vi "外观 1.vi"(0 "Data In":T8 caption="数据输入", 2 "Display State In":T6 caption="显示状态输入", 3 "Container State":T7 caption="容器状态") -> (6 "Data Out":T8 caption="数据输出", 7 "Display State Out":T6 caption="显示状态输出", 8 "Action":T5 caption="动作")   [LabVIEW 2013, in "Bit by Bit Adjust_Xcontrol.xctl"]
uses:
  Bit by Bit Adjust_Xcontrol.xctl
  <vilib>/_xctls/Container State.ctl
  <vilib>/_xctls/Action.ctl
  Bit_Display.ctl
  Up_Key.ctl
  Down_Key.ctl
  %_Display.ctl
  <vilib>/_xctls/XControlSupport.lvlib
panel:
  out "Totol Number":i32
  in  "Zero":bool
  out "小数点":bool=TRUE
  out "字符串":T1="%"
  in  "Down_x1":T2
  in  "Down_x10":T2
  in  "Down_x100":T2
  in  "Down_x1000":T2
  in  "Up_x1":T3
  in  "Up_x10":T3
  in  "Up_x100":T3
  in  "Up_x1000":T3
  out "Str_x1":T4="0"
  out "Str_x10":T4="0"
  out "Str_x100":T4="0"
  out "Str_x1000":T4="0"
  in  "Down_x10000":T2
  in  "Up_x10000":T3
  out "Str_x10000":T4="0"
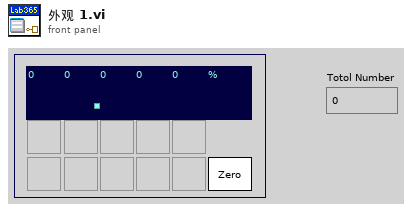
[diagram p1: front panel]
types:
  T1 = typedef "%_Display.ctl" = string
  T2 = typedef "Down_Key.ctl" = bool
  T3 = typedef "Up_Key.ctl" = bool
  T4 = typedef "Bit_Display.ctl" = string
  T5 = typedef "XControlSupport.lvlib/Action.ctl" = cluster{"Data Changed?":bool, "State Changed?":bool, "Action Name":string}
  T6 = typedef "Bit by Bit Adjust_Xcontrol.xctl/状态 1.ctl" = cluster{"Numeric":dbl}
  T7 = typedef "XControlSupport.lvlib/Container State.ctl" = cluster{"Indicator?":bool, "Run Mode?":bool, " Refnum":refnum<vi>}
  T8 = typedef "Bit by Bit Adjust_Xcontrol.xctl/数据 1.ctl" = dbl
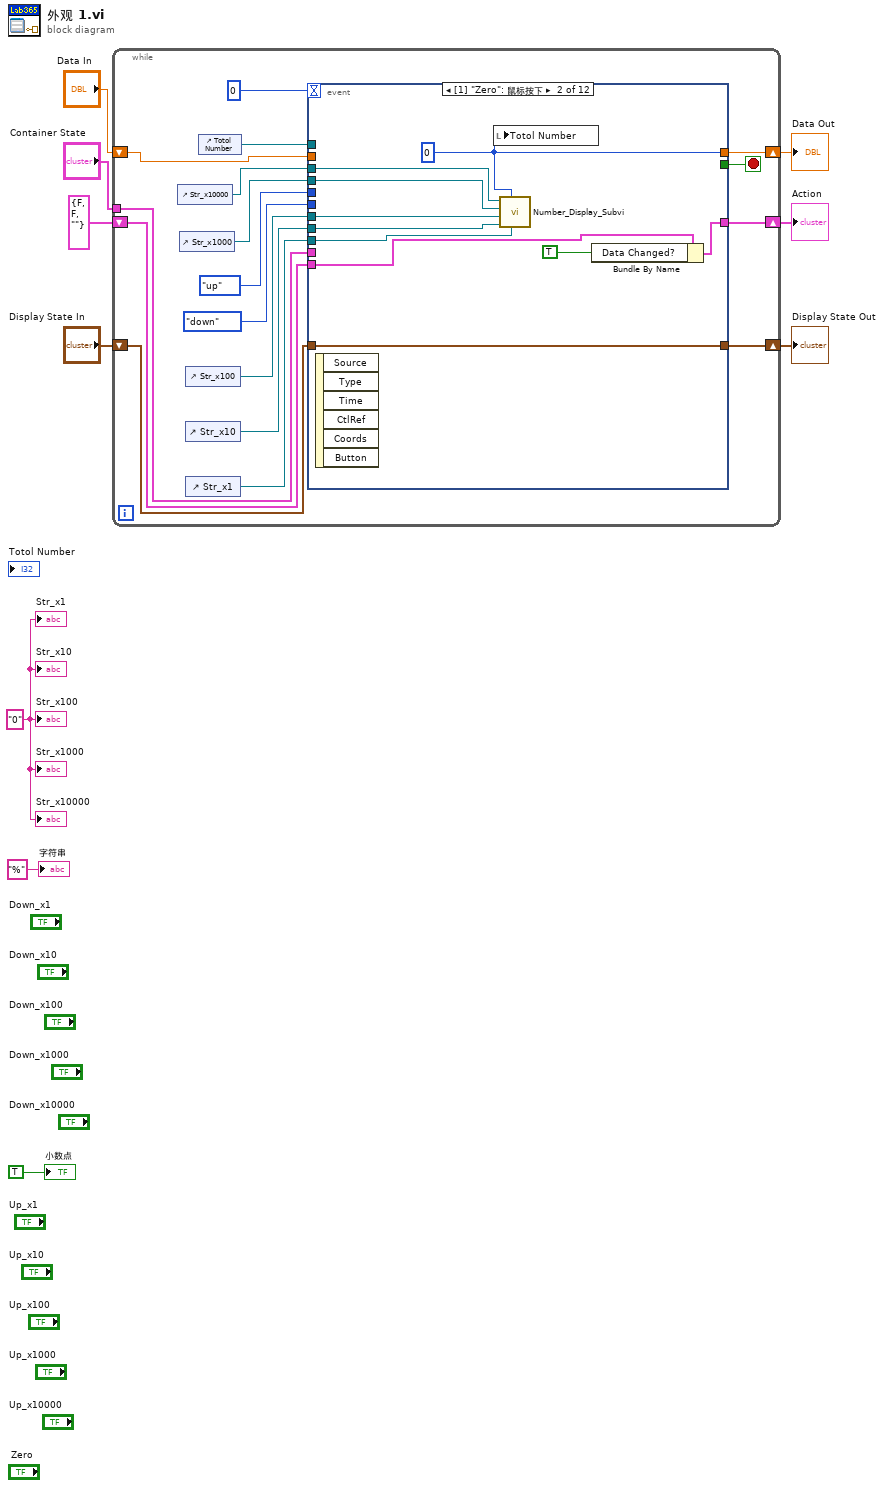
[diagram p0: block diagram]
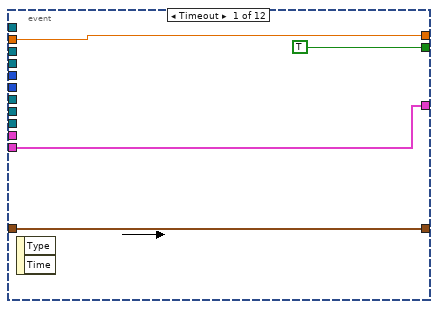
[diagram p2: hidden frame]
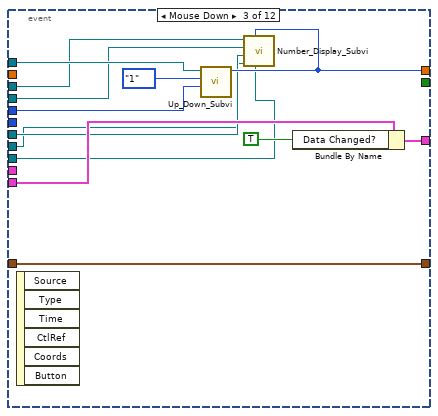
[diagram p3: hidden frame]
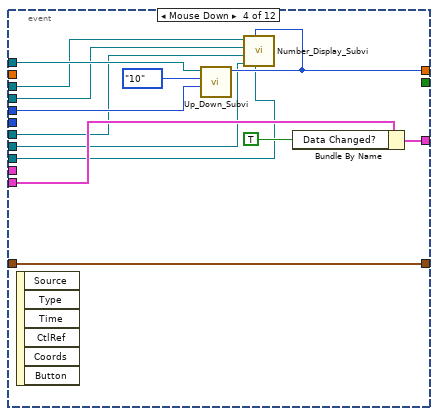
[diagram p4: hidden frame]
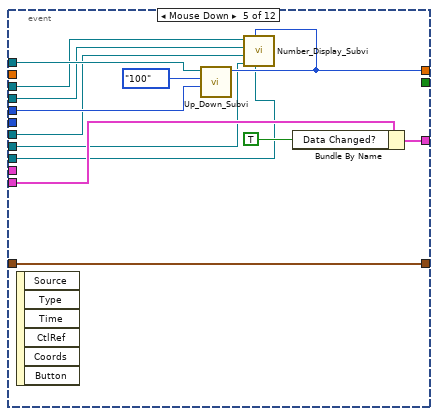
[diagram p5: hidden frame]
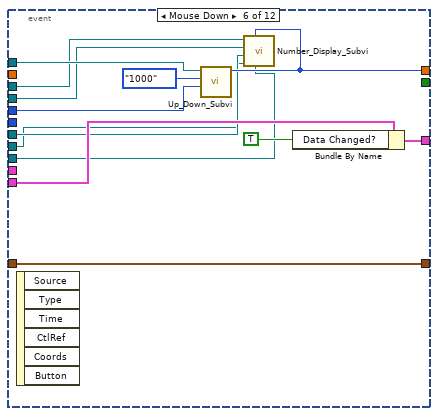
[diagram p6: hidden frame]
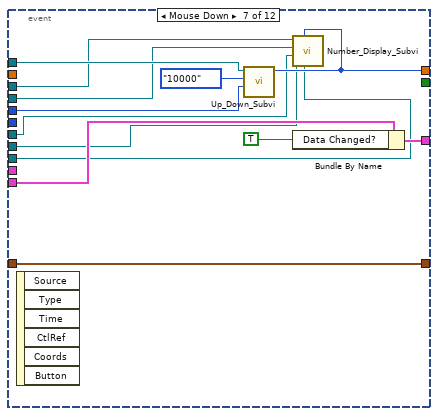
[diagram p7: hidden frame]
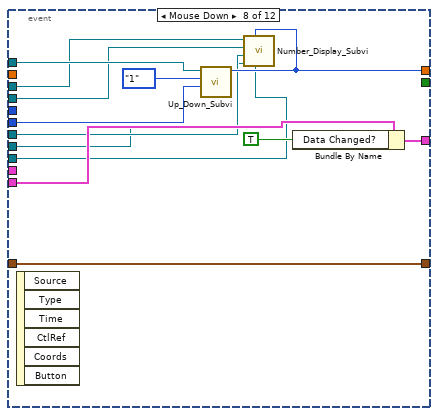
[diagram p8: hidden frame]
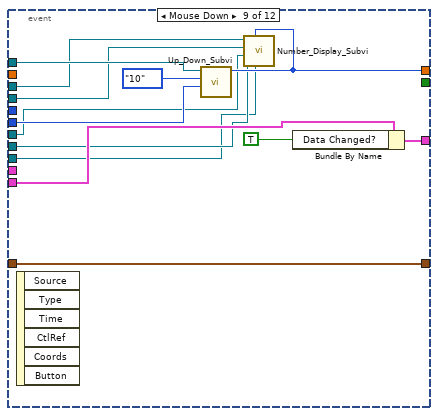
[diagram p9: hidden frame]
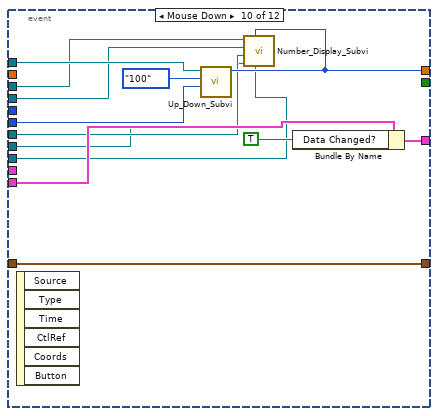
[diagram p10: hidden frame]
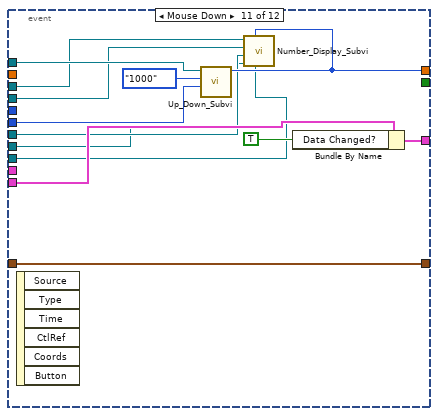
[diagram p11: hidden frame]
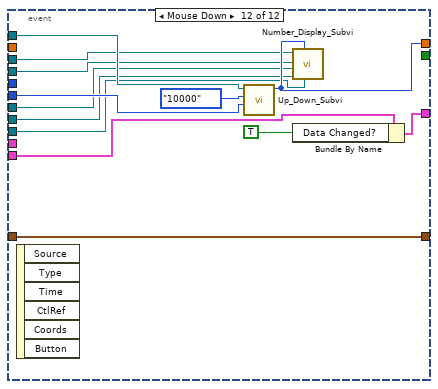
[diagram p12: hidden frame]
diagram:
  w8 = T4 "0" ("数值 5")
  n1 = while {
    shift-right: [w26] -> w4
    shift-left: "Display State In" -> [w27]
    tunnel: "Container State" -> [w23]
    shift-right: [w19] -> w7
    shift-left: "Data In" -> [w22]
    shift-right: [w20] -> w2
    shift-left: T5 {"Data Changed?"=FALSE, "State Changed?"=FALSE, "Action Name"=""} ("Action") -> [w21]
    stop <- w25 stop-if-true
    n2 = control-ref of="Str_x10000"() -> (w15:refnum<vi>)
    n3 = control-ref of="Str_x1000"() -> (w14:refnum<vi>)
    n4 = control-ref of="Str_x100"() -> (w13:refnum<vi>)
    n5 = control-ref of="Str_x10"() -> (w12:refnum<vi>)
    n6 = control-ref of="Str_x1"() -> (w11:refnum<vi>)
    n7 = control-ref of="Totol Number"() -> (w18:refnum<vi>)
    n8 = event shown="[1] \"Zero\": 鼠标按下" {
      selector: _ -> [_ _ _ _ _ _ _ _ _ _ _ _]
      dyn-events: _ -> [_ _ _ _ _ _ _ _ _ _ _ _]
      timeout: 0 -> [_ _ _ _ _ _ _ _ _ _ _ _]
      tunnel: w27 -> [w29 w38 w50 w63 w76 w93 w106 w119 w132 w143 w156 w169]
      tunnel: [w29 w38 w50 w63 w76 w93 w106 w119 w132 w143 w156 w169] -> w26
      tunnel: [TRUE _ _ _ _ _ _ _ _ _ _ _] -> w25
      tunnel: w23 -> [_ _ _ _ _ _ _ _ _ _ _ _]
      tunnel: w22 -> [w28 _ _ _ _ _ _ _ _ _ _ _]
      tunnel: [w28 w37 w47 w60 w73 w86 w99 w112 w125 w138 w151 w164] -> w19
      tunnel: [w30 w40 w51 w65 w78 w91 w104 w115 w130 w140 w154 w167] -> w20
      tunnel: w21 -> [w30 w41 w53 w66 w79 w92 w105 w116 w131 w142 w155 w168]
      tunnel: w18 -> [_ _ w54 w67 w80 w89 w102 w118 w127 w145 w158 w171]
      tunnel: enum16{"up", "down"}."up" ("枚举") -> [_ _ w49 w62 w75 w88 w101 _ _ _ _ _]
      tunnel: enum16{"up", "down"}."down" ("枚举") -> [_ _ _ _ _ _ _ w117 w128 w144 w157 w170]
      tunnel: w15 -> [_ w36 w46 w59 w72 w85 w98 w111 w124 w137 w150 w163]
      tunnel: w14 -> [_ w35 w45 w58 w71 w84 w97 w110 w123 w136 w149 w162]
      tunnel: w13 -> [_ w34 w44 w57 w70 w83 w96 w109 w122 w135 w148 w161]
      tunnel: w12 -> [_ w33 w43 w56 w69 w82 w95 w108 w121 w134 w147 w160]
      tunnel: w11 -> [_ w32 w42 w55 w68 w81 w94 w107 w120 w133 w146 w159]
      event Timeout {
        n9 = event-data() -> ()  [unwired: 3 out]
      }
      event "Zero": Mouse Down {
        w37 = 0 ("总数值")
        n10 = event-data() -> ()  [unwired: 7 out]
        n11 = local write "Totol Number"(w37) -> ()
        n12 = call "Number_Display_Subvi.vi"("Str_x1"=w32, "Totol Number"=w37, "Str_10"=w33, "Str_x100"=w34, "Str_x1000"=w35, "Str_x10000"=w36) -> ()  [unwired: 1 in, 5 out]
        n13 = Bundle By Name(cluster=w41, "Data Changed?"=TRUE) -> (w40:T5)
      }
      event Mouse Down {
        n14 = event-data() -> ()  [unwired: 7 out]
        n15 = call "Up_Down_Subvi.vi"("Up/Down"=w49, "multiplicator"=enum16{"1", "10", "100", "1000", "10000"}."1", "Ref_Totol Number"=w54) -> ("Totol Number"=w47:i32)  [unwired: 8 out]
        n16 = call "Number_Display_Subvi.vi"("Str_x1"=w42, "Totol Number"=w47, "Str_10"=w43, "Str_x100"=w44, "Str_x1000"=w45, "Str_x10000"=w46) -> ()  [unwired: 6 out]
        n17 = Bundle By Name(cluster=w53, "Data Changed?"=TRUE) -> (w51:T5)
      }
      event Mouse Down {
        n18 = event-data() -> ()  [unwired: 7 out]
        n19 = call "Up_Down_Subvi.vi"("Up/Down"=w62, "multiplicator"=enum16{"1", "10", "100", "1000", "10000"}."10", "Ref_Totol Number"=w67) -> ("Totol Number"=w60:i32)  [unwired: 8 out]
        n20 = call "Number_Display_Subvi.vi"("Str_x1"=w55, "Totol Number"=w60, "Str_10"=w56, "Str_x100"=w57, "Str_x1000"=w58, "Str_x10000"=w59) -> ()  [unwired: 6 out]
        n21 = Bundle By Name(cluster=w66, "Data Changed?"=TRUE) -> (w65:T5)
      }
      event Mouse Down {
        n22 = event-data() -> ()  [unwired: 7 out]
        n23 = call "Up_Down_Subvi.vi"("Up/Down"=w75, "multiplicator"=enum16{"1", "10", "100", "1000", "10000"}."100", "Ref_Totol Number"=w80) -> ("Totol Number"=w73:i32)  [unwired: 8 out]
        n24 = call "Number_Display_Subvi.vi"("Str_x1"=w68, "Totol Number"=w73, "Str_10"=w69, "Str_x100"=w70, "Str_x1000"=w71, "Str_x10000"=w72) -> ()  [unwired: 6 out]
        n25 = Bundle By Name(cluster=w79, "Data Changed?"=TRUE) -> (w78:T5)
      }
      event Mouse Down {
        n26 = event-data() -> ()  [unwired: 7 out]
        n27 = call "Up_Down_Subvi.vi"("Up/Down"=w88, "multiplicator"=enum16{"1", "10", "100", "1000", "10000"}."1000", "Ref_Totol Number"=w89) -> ("Totol Number"=w86:i32)  [unwired: 8 out]
        n28 = call "Number_Display_Subvi.vi"("Str_x1"=w81, "Totol Number"=w86, "Str_10"=w82, "Str_x100"=w83, "Str_x1000"=w84, "Str_x10000"=w85) -> ()  [unwired: 6 out]
        n29 = Bundle By Name(cluster=w92, "Data Changed?"=TRUE) -> (w91:T5)
      }
      event Mouse Down {
        n30 = event-data() -> ()  [unwired: 7 out]
        n31 = call "Up_Down_Subvi.vi"("Up/Down"=w101, "multiplicator"=enum16{"1", "10", "100", "1000", "10000"}."10000", "Ref_Totol Number"=w102) -> ("Totol Number"=w99:i32)  [unwired: 8 out]
        n32 = call "Number_Display_Subvi.vi"("Str_x1"=w94, "Totol Number"=w99, "Str_10"=w95, "Str_x100"=w96, "Str_x1000"=w97, "Str_x10000"=w98) -> ()  [unwired: 6 out]
        n33 = Bundle By Name(cluster=w105, "Data Changed?"=TRUE) -> (w104:T5)
      }
      event Mouse Down {
        n34 = event-data() -> ()  [unwired: 7 out]
        n35 = call "Up_Down_Subvi.vi"("Up/Down"=w117, "multiplicator"=enum16{"1", "10", "100", "1000", "10000"}."1", "Ref_Totol Number"=w118) -> ("Totol Number"=w112:i32)  [unwired: 8 out]
        n36 = call "Number_Display_Subvi.vi"("Str_x1"=w107, "Totol Number"=w112, "Str_10"=w108, "Str_x100"=w109, "Str_x1000"=w110, "Str_x10000"=w111) -> ()  [unwired: 6 out]
        n37 = Bundle By Name(cluster=w116, "Data Changed?"=TRUE) -> (w115:T5)
      }
      event Mouse Down {
        n38 = event-data() -> ()  [unwired: 7 out]
        n39 = call "Up_Down_Subvi.vi"("Up/Down"=w128, "multiplicator"=enum16{"1", "10", "100", "1000", "10000"}."10", "Ref_Totol Number"=w127) -> ("Totol Number"=w125:i32)  [unwired: 8 out]
        n40 = call "Number_Display_Subvi.vi"("Str_x1"=w120, "Totol Number"=w125, "Str_10"=w121, "Str_x100"=w122, "Str_x1000"=w123, "Str_x10000"=w124) -> ()  [unwired: 6 out]
        n41 = Bundle By Name(cluster=w131, "Data Changed?"=TRUE) -> (w130:T5)
      }
      event Mouse Down {
        n42 = event-data() -> ()  [unwired: 7 out]
        n43 = call "Up_Down_Subvi.vi"("Up/Down"=w144, "multiplicator"=enum16{"1", "10", "100", "1000", "10000"}."100", "Ref_Totol Number"=w145) -> ("Totol Number"=w138:i32)  [unwired: 8 out]
        n44 = call "Number_Display_Subvi.vi"("Str_x1"=w133, "Totol Number"=w138, "Str_10"=w134, "Str_x100"=w135, "Str_x1000"=w136, "Str_x10000"=w137) -> ()  [unwired: 6 out]
        n45 = Bundle By Name(cluster=w142, "Data Changed?"=TRUE) -> (w140:T5)
      }
      event Mouse Down {
        n46 = event-data() -> ()  [unwired: 7 out]
        n47 = call "Up_Down_Subvi.vi"("Up/Down"=w157, "multiplicator"=enum16{"1", "10", "100", "1000", "10000"}."1000", "Ref_Totol Number"=w158) -> ("Totol Number"=w151:i32)  [unwired: 8 out]
        n48 = call "Number_Display_Subvi.vi"("Str_x1"=w146, "Totol Number"=w151, "Str_10"=w147, "Str_x100"=w148, "Str_x1000"=w149, "Str_x10000"=w150) -> ()  [unwired: 6 out]
        n49 = Bundle By Name(cluster=w155, "Data Changed?"=TRUE) -> (w154:T5)
      }
      event Mouse Down {
        n50 = event-data() -> ()  [unwired: 7 out]
        n51 = call "Up_Down_Subvi.vi"("Up/Down"=w170, "multiplicator"=enum16{"1", "10", "100", "1000", "10000"}."10000", "Ref_Totol Number"=w171) -> ("Totol Number"=w164:i32)  [unwired: 8 out]
        n52 = call "Number_Display_Subvi.vi"("Str_x1"=w159, "Totol Number"=w164, "Str_10"=w160, "Str_x100"=w161, "Str_x1000"=w162, "Str_x10000"=w163) -> ()  [unwired: 6 out]
        n53 = Bundle By Name(cluster=w168, "Data Changed?"=TRUE) -> (w167:T5)
      }
    }
  }
  "Display State Out" <- w4
  "Data Out" <- w7
  "Action" <- w2
  "Str_x1000" <- w8
  "Str_x100" <- w8
  "Str_x10" <- w8
  "Str_x1" <- w8
  "Str_x10000" <- w8
  "字符串" <- T1 "%" ("字符串")
  "小数点" <- TRUE ("小数点")
